vi "Path Notation End Name.vi"(11 "Item Path":string) -> (2 "<JSON>End Names":string[](array[string]))   [LabVIEW 2015, in "JSONtext.lvlib"]
uses:
  JSONtext.lvlib
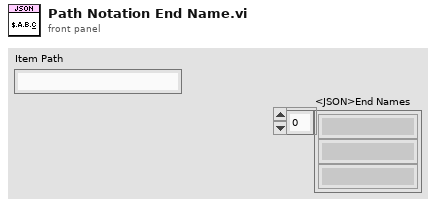
[diagram p1: front panel]
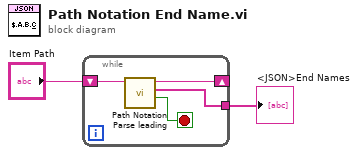
[diagram p0: block diagram]
diagram:
  n1 = while {
    shift-right: [w5] -> _
    shift-left: "Item Path" -> [w6]
    tunnel: [w4] -> w1
    stop <- w3 stop-if-true
    n2 = call "Path Notation Parse leading.vi"("Item Path"=w6) -> ("End of Path"=w3:bool, "<JSON>element names"=w4:string[], "Rest of Path"=w5:string)  [unwired: 8 in]
  }
  "<JSON>End Names" <- w1
